vi "Run.vi"(8 "error in (no error)":errorcluster, 11 "Simulation Interface in":refnum<class "Simulation Interface.lvclass">) -> (0 "error out":errorcluster, 3 "Simulation Interface out":refnum<class "Simulation Interface.lvclass">)   [LabVIEW 2016, in "Simulation Interface.lvclass"]
uses:
  Simulation Interface.lvclass
  Car Wash Controller/Car Wash Controller.lvclass
  Entry Console/Entry Console.lvclass
  Vehicle Position Simulation/Vehicle Position Simulation.lvclass
  Wash Display Console/Wash Display Console.lvclass
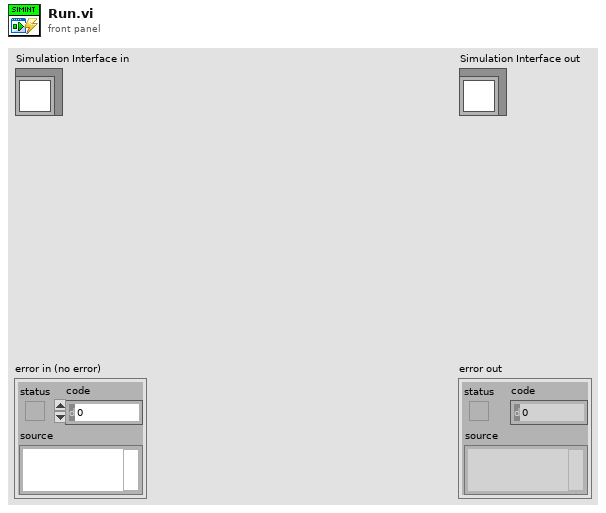
[diagram p1: front panel]
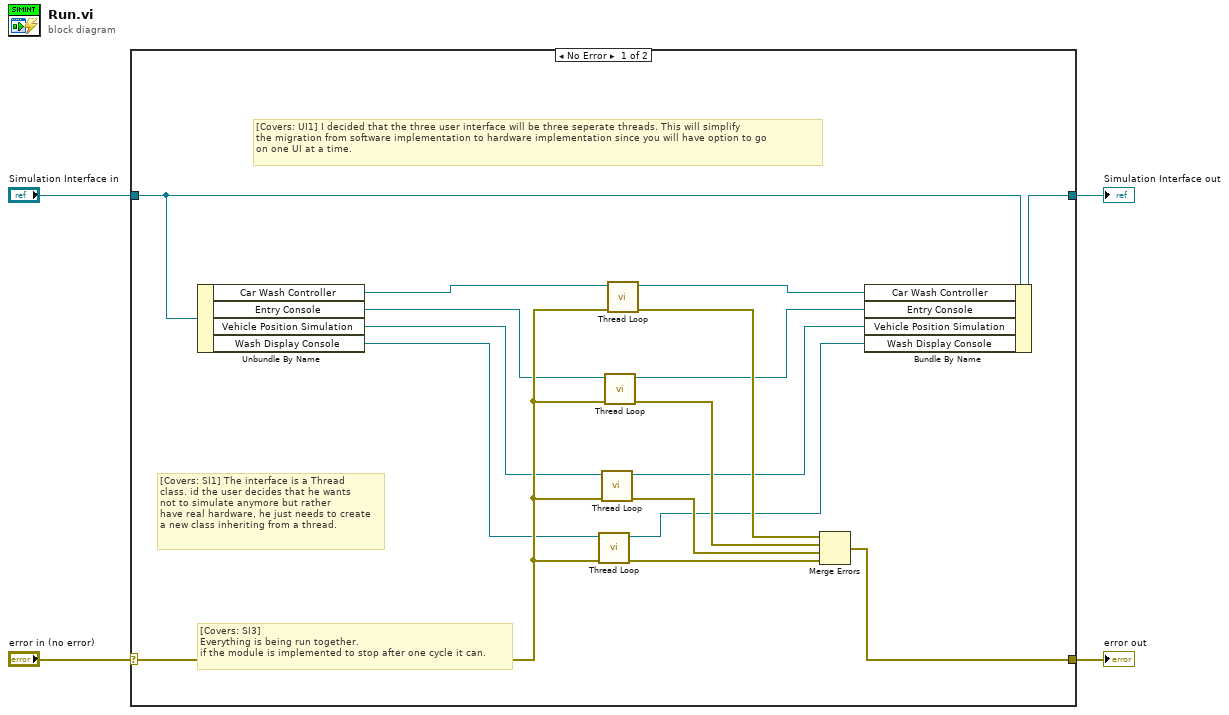
[diagram p0: block diagram]
diagram:
  n1 = case shown="No Error" "error in (no error)" {
    selector: "error in (no error)" -> [w16 w22]
    tunnel: [w15 w22] -> w3
    tunnel: [w9 w21] -> w1
    tunnel: "Simulation Interface in" -> [w10 w21]
    frame No Error {
      # "[Covers: UI1] I decided that the three user interface will be three seperate threads. This will simplify\nthe migration from software implementation to hardware implementation since you will have option to go \non one UI at a time."
      # "[Covers: SI3]\nEverything is being run together.\nif the module is implemented to stop after one cycle it can."
      # "[Covers: SI1] The interface is a Thread\nclass. id the user decides that he wants \nnot to simulate anymore but rather \nhave real hardware, he just needs to create\na new class inheriting from a thread."
      n2 = Unbundle By Name(w10) -> ("Car Wash Controller"=w14:refnum<class "Car Wash Controller.lvclass">, "Entry Console"=w13:refnum<class "Entry Console.lvclass">, "Vehicle Position Simulation"=w12:refnum<class "Vehicle Position Simulation.lvclass">, "Wash Display Console"=w11:refnum<class "Wash Display Console.lvclass">)
      n3 = call-dynamic "Thread Loop.vi"("error in (no error)"=w16, "Wash Display Console in"=w11) -> ("error out"=w17:errorcluster, "Wash Display Console out"=w5:refnum<class "Wash Display Console.lvclass">)  [unwired: 8 in]
      n4 = call-dynamic "Thread Loop.vi"("error in (no error)"=w16, "Vehicle Position Simulation in"=w12) -> ("error out"=w18:errorcluster, "Vehicle Position Simulation out"=w6:refnum<class "Vehicle Position Simulation.lvclass">)  [unwired: 8 in]
      n5 = call-dynamic "Thread Loop.vi"("error in (no error)"=w16, "Entry Console in"=w13) -> ("error out"=w19:errorcluster, "Entry Console out"=w7:refnum<class "Entry Console.lvclass">)  [unwired: 8 in]
      n6 = call-dynamic "Thread Loop.vi"("error in (no error)"=w16, "Car Wash Controller in"=w14) -> ("error out"=w20:errorcluster, "Car Wash Controller out"=w8:refnum<class "Car Wash Controller.lvclass">)  [unwired: 8 in]
      n7 = Merge Errors(w20, w19, w18, w17) -> (w15:errorcluster)
      n8 = Bundle By Name(cluster=w10, "Car Wash Controller"=w8, "Entry Console"=w7, "Vehicle Position Simulation"=w6, "Wash Display Console"=w5) -> (w9:refnum<class "Simulation Interface.lvclass">)
    }
    frame Error {
    }
  }
  "error out" <- w3
  "Simulation Interface out" <- w1
